vi "AudioPlayer.vi"() -> ()   [LabVIEW 2011]
uses:
  <vilib>/sound/lvsound.llb/Sound Format.ctl
  AudioGlobal.vi
  <vilib>/Analysis/2dsp.llb/Resample (constant to constant,single -channel).vi
  <vilib>/Analysis/baseanly.llb/Scale 1D.vi
  <vilib>/Analysis/NI_AALBase.lvlib
  <vilib>/Analysis/NI_AALPro.lvlib
panel:
  in  "Trace to play":i32
  in  "playbackSpeed":dbl(slide)=1.0 min=0.1 max=10.0 step=0.1 scale=0.1..10.0
  in  "fs":dbl=5000.0
  out "TimeTraces":dbl[](graph)
  in  "amplitudeScaling":i16=30000
  out "error out":errorcluster
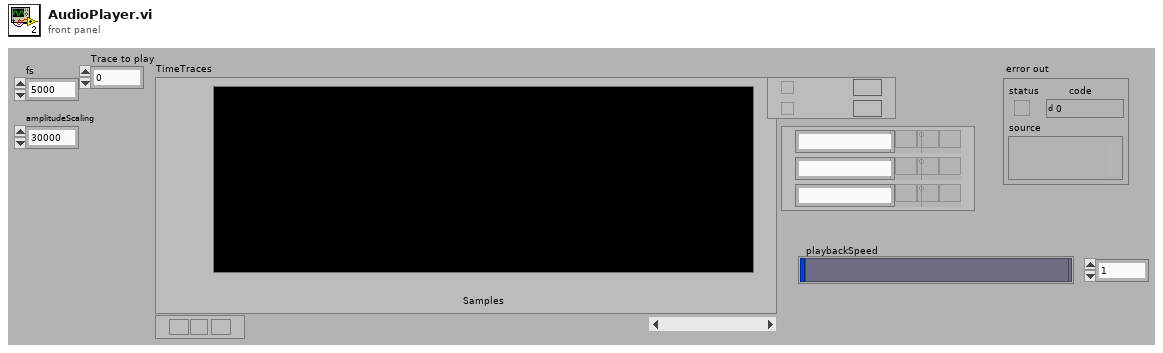
[diagram p1: front panel]
types:
  T1 = typedef "Sound Format.ctl" = cluster{"sound quality":enum16{"mono", "stereo"}, "rate":enum16{"11025", "22050", "44100", "8000"}, "bits per sample":enum16{"8 bit", "16 bit"}}
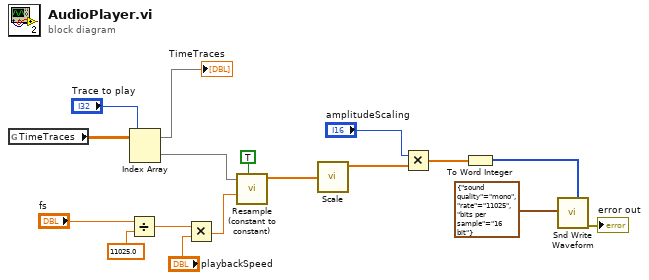
[diagram p0: block diagram]
diagram:
  n1 = global read "AudioGlobal.vi" "TimeTraces"() -> (w4:dbl[][])
  n2 = Divide(x="fs", y=11025.0 ("x")) -> (x/y=w12:dbl)
  n3 = Index Array(array=w4, index (row)="Trace to play") -> (element=w3:dbl[])  [unwired: 1 in]
  "TimeTraces" <- w3
  n4 = Multiply(x=w12, y="playbackSpeed") -> (x*y=w9:dbl)
  n5 = call-poly <vilib>:"Resample (constant to constant).vi"("reset?"=TRUE, "dt"=w9, "X"=w3) -> ("Y"=w2:dbl[])  [unwired: 6 in, 2 out]
  n6 = call-poly <vilib>:"Scale.vi"("X"=w2) -> ("Y=(X-offset)/scale"=w15:dbl[])  [unwired: 3 out]
  n7 = Multiply(x="amplitudeScaling", y=w15) -> (x*y=w13:dbl[])
  n8 = To Word Integer(number=w13) -> (16bit integer=w1:i16[])
  n9 = call <vilib>:"Snd Write Waveform.vi"("mono 16-bit"=w1, "sound format"=T1 {"sound quality"=enum."mono", "rate"=enum."11025", "bits per sample"=enum."16 bit"}) -> ("error out"=→"error out":errorcluster)  [unwired: 9 in]
